vi "4.6.vi"() -> ()   [LabVIEW 2015]
uses:
  <vilib>/Analysis/NI_AALPro.lvlib
panel:
  out "XY Graph":cluster{dbl[], dbl[]}(graph)
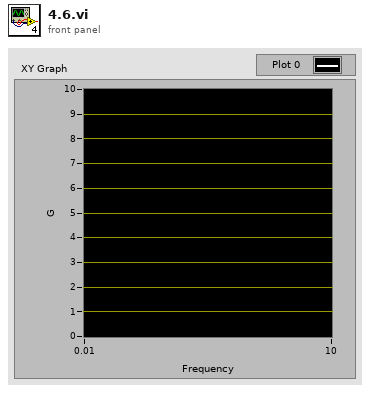
[diagram p1: front panel]
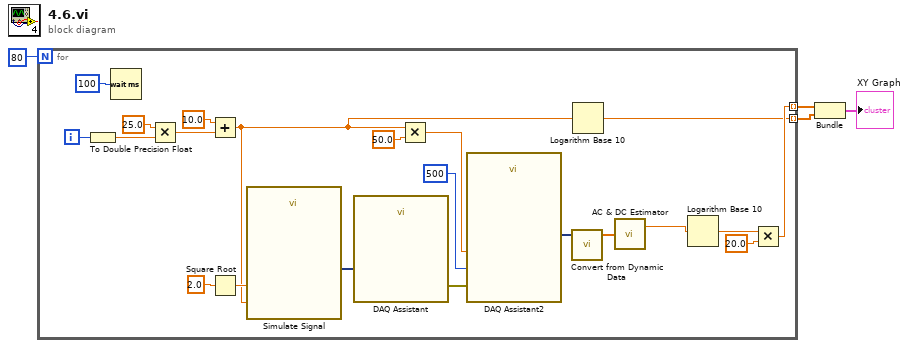
[diagram p0: block diagram]
diagram:
  n1 = for {
    N: 80 -> [_]
    tunnel: [w12] -> w2 mode=indexing
    tunnel: [w11] -> w1 mode=indexing
    i -> [w19]
    n2 = To Double Precision Float(number=w19) -> (double precision float=w18:dbl)
    n3 = Wait (ms)(milliseconds to wait=100) -> ()  [unwired: 1 out]
    n4 = Multiply(x=25.0, y=w18) -> (x*y=w21:dbl)
    n5 = Add(x=10.0, y=w21) -> (x+y=w17:dbl)
    n6 = Square Root(x=2.0) -> (sqrt(x)=w25:dbl)
    n7 = call "Simulate Signal"("Frequency"=w17, "Amplitude"=w25) -> ("Sine"=w10:dynamicdata)  [unwired: 12 in, 1 out]
    n8 = call "DAQ Assistant"("data"=w10) -> ("error out"=w7:errorcluster)  [unwired: 16 in, 2 out]
    n9 = Multiply(x=w17, y=50.0) -> (x*y=w8:dbl)
    n10 = call "DAQ Assistant2"("rate"=w8, "number of samples"=500, "error in"=w7) -> ("data"=w6:dynamicdata)  [unwired: 14 in, 2 out]
    n11 = call "Convert from Dynamic Data"("Dynamic Data Type"=w6) -> ("Array"=w13:dbl[])  [unwired: 3 in]
    n12 = Logarithm Base 10(1:w17) -> (0:w11:dbl)
    n13 = call <vilib>:"AC & DC Estimator.vi"("Signal (V)"=w13) -> ("AC estimate (Vrms)"=w5:dbl)  [unwired: 1 out]
    n14 = Logarithm Base 10(1:w5) -> (0:w16:dbl)
    n15 = Multiply(x=w16, y=20.0) -> (x*y=w12:dbl)
  }
  n16 = Bundle(w2, w1) -> (→"XY Graph":cluster{dbl[], dbl[]})  [unwired: 1 in]
